vi "Evaluate Part 2.vi"() -> ()   [LabVIEW 2020]
uses:
  Proto/NetAn.lvclass
panel:
  out "Answer":string
  in  "Input":string="kh-tc\nqp-kh\nde-cg\nka-co\nyn-aq\nqp-ub\ncg-tb\nvc-aq\ntb-ka\nwh-tc\nyn-cg\nkh-ub\nta-co\nde-co\ntc-td\ntb-wq\nwh-td\nta-ka\ntd-qp\naq-cg\nwq-ub\nub-vc\nde-ta\nwq-aq\nwq-vc\nwh-yn\nka-de\nkh-ta\nco-tc\nwh-qp\ntb-vc\ntd-yn"
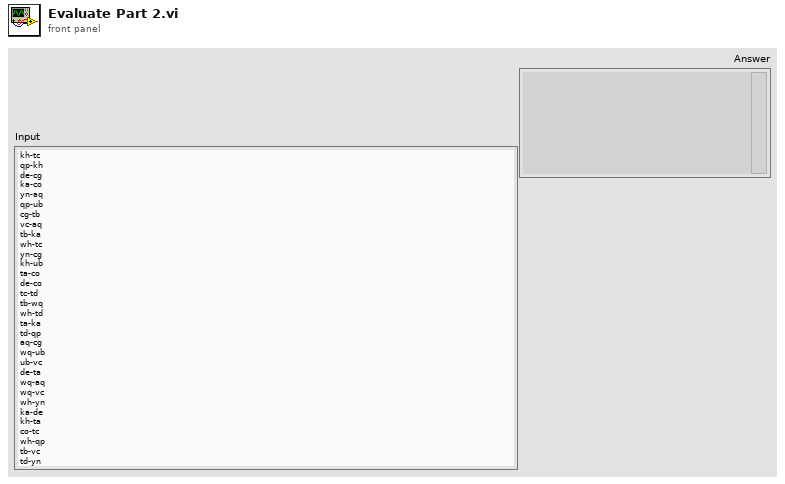
[diagram p1: front panel]
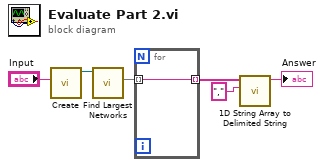
[diagram p0: block diagram]
diagram:
  n1 = call "Create.vi"("Input"="Input") -> ("Proto"=w5:refnum<class "NetAn.lvclass">)  [unwired: 9 in, 1 out]
  n2 = call "Find Largest Networks.vi"("Proto in"=w5) -> ("set"=w4:set{string})  [unwired: 8 in, 2 out]
  n3 = for {
    tunnel: w4 -> [w7] mode=indexing
    tunnel: [w7] -> w3 mode=indexing
  }
  n4 = call <vilib>:"1D String Array to Delimited String.vi"("delimiter"=",", "string array"=w3) -> ("delimited string"=→"Answer":string)  [unwired: 9 in]
